vi "initialize.vi"(8 "error in (no error)":errorcluster, 11 "pdbm_testsys_event":T2) -> (0 "error IO":errorcluster, 2 "pdbm_taskroute_reg_event":T3, 3 "pdbm_taskroute_event":T1)   [LabVIEW 2015, in "pdbm_task_route.lvlib"]
uses:
  pdbm_task_route.lvlib
  pdbm_testsys_taskroute_inter/UsrDefine/pdbm_testsys_reqst_data.ctl
  test_system/UsrDefine/pdbm_testsystem_feedback_data.ctl
  UsrDefine/TaskFeedbackCmd.ctl
  test_system/pdbm_test_system.lvlib
  pdbm_testsys_taskroute_inter/pdbm_testsys_taskroute_inter.lvlib
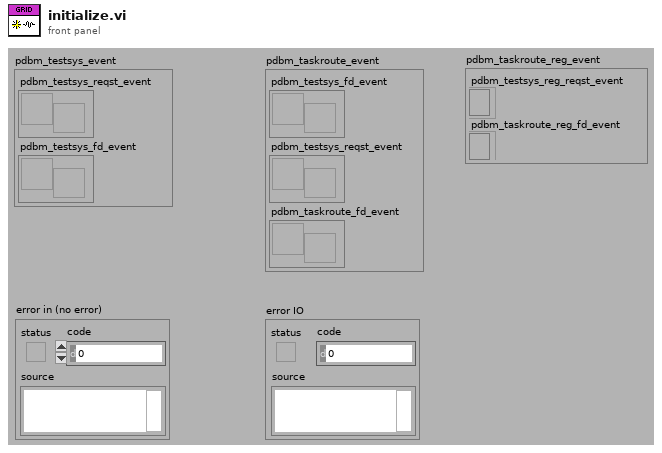
[diagram p1: front panel]
types:
  T1 = cluster{"pdbm_testsys_fd_event":refnum<user-event>, "pdbm_testsys_reqst_event":refnum<user-event>, "pdbm_taskroute_fd_event":refnum<user-event>}
  T2 = cluster{"pdbm_testsys_reqst_event":refnum<user-event>, "pdbm_testsys_fd_event":refnum<user-event>}
  T3 = cluster{"pdbm_testsys_reg_reqst_event":refnum<event-registration>, "pdbm_taskroute_reg_fd_event":refnum<event-registration>}
  T4 = cluster{"pdbm_testsys_fd_event":refnum<user-event>, "pdbm_testsys_reqst_event":refnum<user-event>, "pdbm_task_fb_info_queue":refnum<user-event>}
  T5 = cluster{"Event Registration Refnum":refnum<event-registration>, "Event Registration Refnum":refnum<event-registration>}
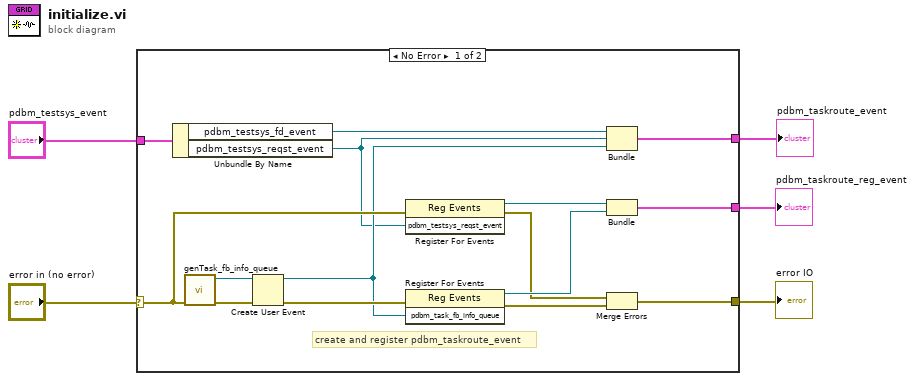
[diagram p0: block diagram]
diagram:
  n1 = case shown="No Error" "error in (no error)" {
    selector: "error in (no error)" -> [w11 w21]
    tunnel: [w15 w21] -> w4
    tunnel: [w12 _] -> w3
    tunnel: "pdbm_testsys_event" -> [w9 _]
    tunnel: [w6 _] -> w1
    frame No Error {
      # "create and register pdbm_taskroute_event"
      n2 = Unbundle By Name(w9) -> ("pdbm_testsys_fd_event"=w7:refnum<user-event>, "pdbm_testsys_reqst_event"=w8:refnum<user-event>)
      n3 = call "genTask_fb_info_queue.vi"("error in (no error)"=w11) -> ("error IO"=w19:errorcluster, "pdbm_task_fb_info_queue"=w20:refnum<queue>)  [unwired: 9 in]
      n4 = Create User Event(user event datatype=w20, error in=w19) -> (user event=w10:refnum<user-event>, error out=w18:errorcluster)
      n5 = register-events(error in=w11, w8) -> (reference out=w17:refnum<event-registration>, error out=w13:errorcluster)  [unwired: 1 in]
      n6 = register-events(error in=w18, w10) -> (reference out=w16:refnum<event-registration>, error out=w14:errorcluster)  [unwired: 1 in]
      n7 = Bundle("pdbm_testsys_fd_event"=w7, "pdbm_testsys_reqst_event"=w8, "pdbm_task_fb_info_queue"=w10) -> (w6:T4)  [unwired: 1 in]
      n8 = Bundle("Event Registration Refnum"=w17, "Event Registration Refnum"=w16) -> (w12:T5)  [unwired: 1 in]
      n9 = Merge Errors(w13, w14) -> (w15:errorcluster)
    }
    frame Error {
    }
  }
  "error IO" <- w4
  "pdbm_taskroute_reg_event" <- w3
  "pdbm_taskroute_event" <- w1
